vi "Write Configuration.vi"(6 "Array":dbl[][](array[numeric]), 8 "Real Matrix":T1, 9 "Configuration":T2={"Accelerometer Bias"={"X (m/s)"=0.0, "Y (m/s)"=0.0, "Z (m/s)"=0.0}, "Gyroscope Bias"={"X (m/s)"=0.0, "Y (m/s)"=0.0, "Z (m/s)"=0.0}, "Steering Motor Gear Ratio"=611.0, "Steering Pully Gear Ratio"=1.0, "Steering Encoder CPR"=500.0, "Steering Motor Max RPM"=4000.0, "Wheelbase (m)"=1.12, "Fork Angle (rad)"=1.3, "Balancing Controller"={"Kp (/s)"=0.0, "Kd (1)"=0.0}, "Max Allowed Steering Angle (rad)"=0.7, "Task Periods"={"Emergency Stop (us)"=0, "IMU (us)"=0, "Steering Motor Encoder (us)"=0, "State Estimator (us)"=0, "Balancing Controller (us)"=0, "GNSS (us)"=0, "Logging (us)"=0, "Drive Motor (us)"=0, "Visualization (us)"=50000}, "Drive Motor Gear Ratio"=0.7, "lr"=0.0, "lf"=0.0, "lambda"=0.0, "k1"=0.0, "k2"=0.0, "e1_max"=0.0, "Ad_tmin"=0.0, "Bd_tmin"=0.0, "C_tmin"=0.0, "D_tmin"=0.0, "Wheel radius"=0.311, "Ad_tmax"=0.95971, "Bd_tmax"=0.01, "C_tmax"=2.20588, "D_tmax"=0.0, "Vmin"=2.20588, "Vmax"=0.0}, 10 "XML File Path conf":path=path "c:/ni-rt/startup/configuration.xml", 11 "Error In":errorcluster) -> (3 "Error Out":errorcluster)   [LabVIEW 2021]
uses:
  Configuration.ctl
  <vilib>/Analysis/Matrix/Datatypes/RealMatrix.ctl
  <vilib>/Utility/xml.llb/Write to XML File(string).vi
  <vilib>/Analysis/Matrix/NI_Matrix.lvlib
panel:
  out "error out 2":errorcluster
  in  "error in (no error) 2":errorcluster
  in  "XML File Path matr 2":path=path "c:/ni-rt/startup/trajectorylab.xml"
  out "error out":errorcluster
  in  "error in (no error)":errorcluster
  in  "XML File Path matr":path=path "c:/ni-rt/startup/matrixlab.xml"
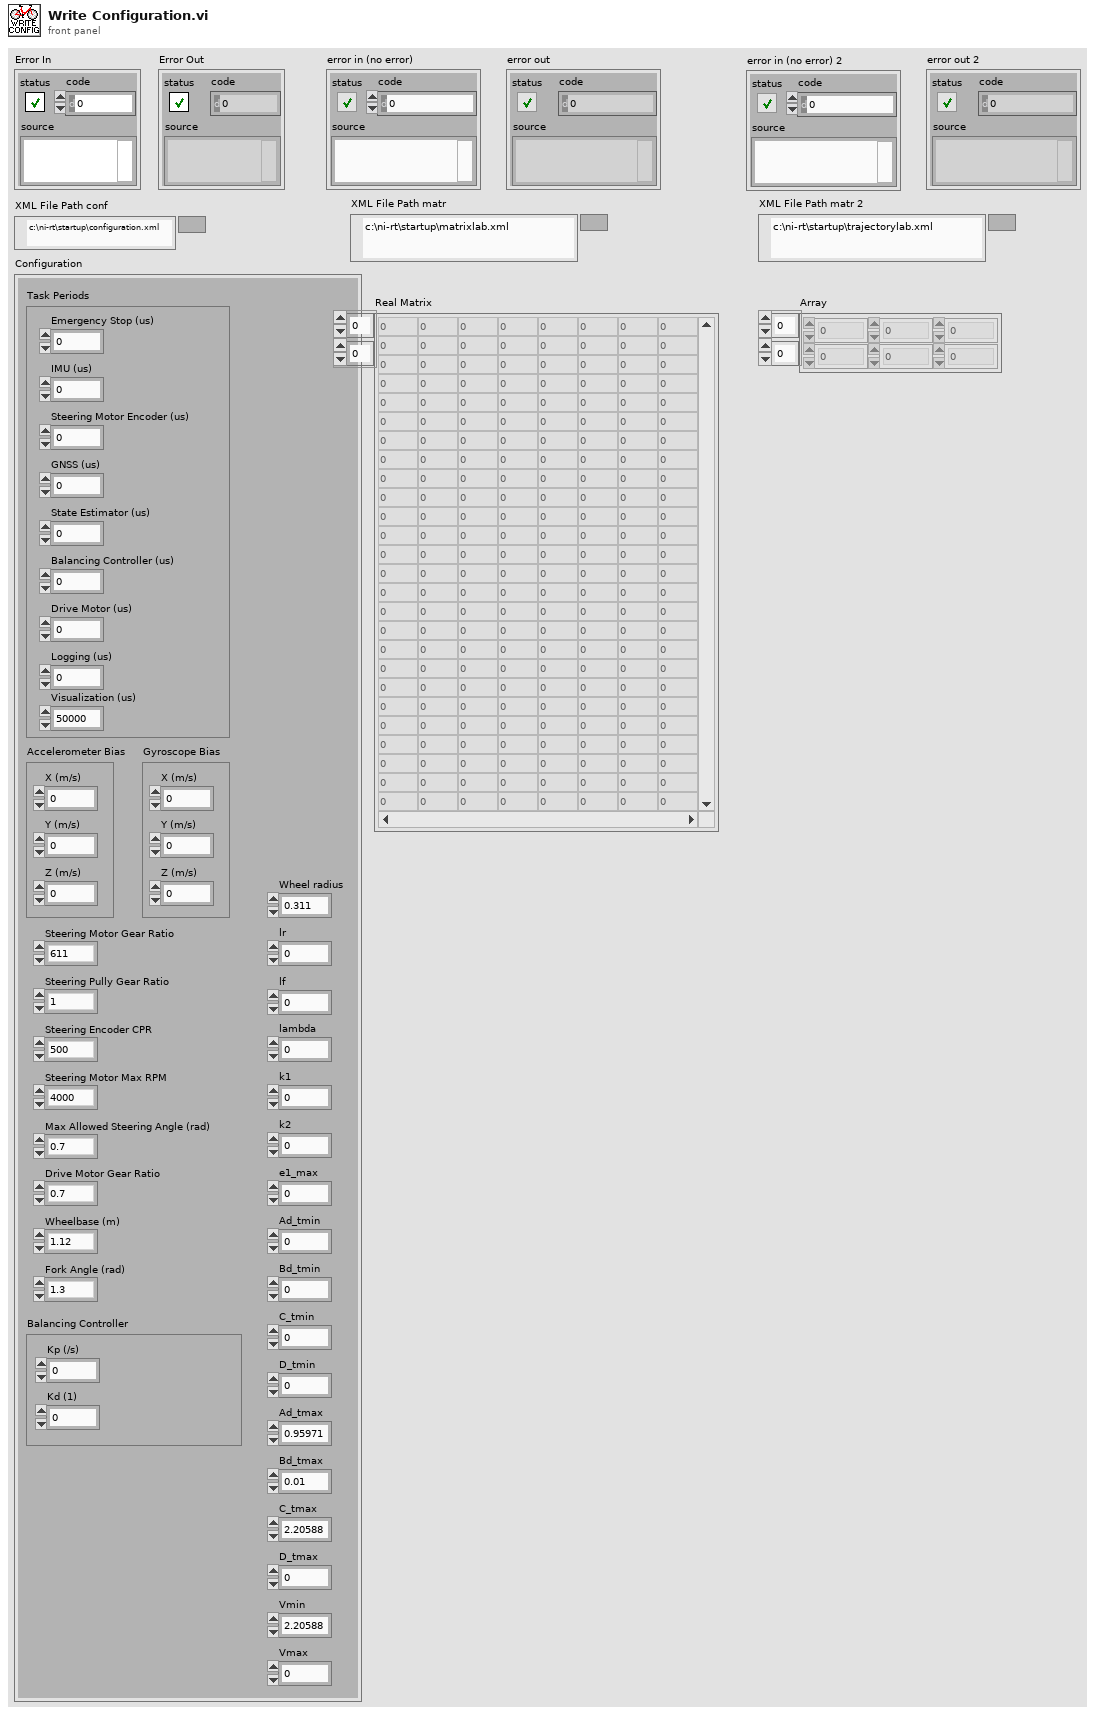
[diagram p1: front panel]
types:
  T1 = typedef "NI_Matrix.lvlib/RealMatrix.ctl" = dbl[][]
  T2 = typedef "Configuration.ctl" = cluster{"Accelerometer Bias":cluster{"X (m/s)":dbl, "Y (m/s)":dbl, "Z (m/s)":dbl}, "Gyroscope Bias":cluster{"X (m/s)":dbl, "Y (m/s)":dbl, "Z (m/s)":dbl}, "Steering Motor Gear Ratio":dbl, "Steering Pully Gear Ratio":dbl, "Steering Encoder CPR":dbl, "Steering Motor Max RPM":dbl, "Wheelbase (m)":dbl, "Fork Angle (rad)":dbl, "Balancing Controller":cluster{"Kp (/s)":dbl, "Kd (1)":dbl}, "Max Allowed Steering Angle (rad)":dbl, "Task Periods":cluster{"Emergency Stop (us)":i64, "IMU (us)":i64, "Steering Motor Encoder (us)":i64, "State Estimator (us)":i64, "Balancing Controller (us)":i64, "GNSS (us)":i64, "Logging (us)":i64, "Drive Motor (us)":i64, "Visualization (us)":i64}, "Drive Motor Gear Ratio":dbl, "lr":dbl, "lf":dbl, "lambda":dbl, "k1":dbl, "k2":dbl, "e1_max":dbl, "Ad_tmin":dbl, "Bd_tmin":dbl, "C_tmin":dbl, "D_tmin":dbl, "Wheel radius":dbl, "Ad_tmax":dbl, "Bd_tmax":dbl, "C_tmax":dbl, "D_tmax":dbl, "Vmin":dbl, "Vmax":dbl}
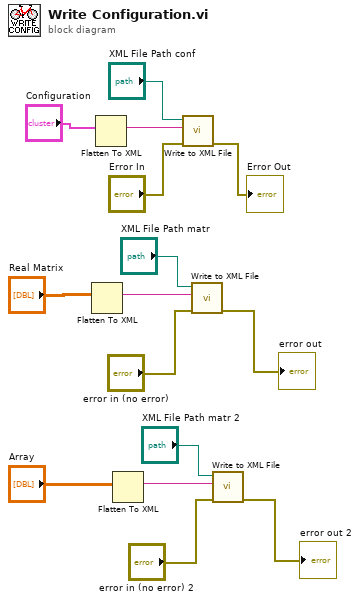
[diagram p0: block diagram]
diagram:
  n1 = Flatten To XML(6:"Real Matrix") -> (2:w10:string)
  n2 = Flatten To XML(6:"Configuration") -> (2:w15:string)
  n3 = Flatten To XML(6:"Array") -> (2:w6:string)
  n4 = call-poly <vilib>:"Write to XML File.vi"("error in (no error)"="Error In", "XML Input"=w15, "XML File Path"="XML File Path conf") -> ("error out"=→"Error Out":errorcluster)  [unwired: 6 in, 2 out]
  n5 = call-poly <vilib>:"Write to XML File.vi"("error in (no error)"="error in (no error)", "XML Input"=w10, "XML File Path"="XML File Path matr") -> ("error out"=→"error out":errorcluster)  [unwired: 6 in, 2 out]
  n6 = call-poly <vilib>:"Write to XML File.vi"("error in (no error)"="error in (no error) 2", "XML Input"=w6, "XML File Path"="XML File Path matr 2") -> ("error out"=→"error out 2":errorcluster)  [unwired: 6 in, 2 out]
